vi "After Launch Init.vi"(8 "error in (no error)":errorcluster, 11 "CS++DCPwr in":refnum<class "CS++DCPwr.lvclass">) -> (0 "error out":errorcluster, 3 "CS++DCPwr out":refnum<class "CS++DCPwr.lvclass">)   [LabVIEW 2013, in "CS++DCPwr.lvlib" / "CS++DCPwr.lvclass"]
doc: "Use <b>Pre Launch init.vi</b> method for sanity checks that are supposed to prevent the actor from launching if they fail. Use <B>this</B> method instead to initialize this actor when it has been activated. A corresponding high priority message will become dispatched before the <B>Actor Core.vi</b> is called.\n\nRefer also to the ongoing discussion at https://decibel.ni.com/content/message/57394#57394."
uses:
  CS++DCPwr.lvclass
  Core/Classes/CS++ProcessVariables/SVConnection/SVConnection.lvclass
  CS++DCPwr.lvclass/CS++DCPwr.ctl
  Core/Classes/CS++ProcessVariables/PVConnection/PVConnection.lvclass/PVConnection.ctl
  Core/Actors/CS++DeviceActor/CS++DeviceActor.lvclass
  Core/Actors/CS++DeviceActor/CS++DeviceActor.lvclass/CS++DeviceActor.ctl
  CS++DCPwr Messages/Measure [MSR] Msg/Measure [MSR] Msg.lvclass
  <vilib>/ActorFramework/Actor/Actor.lvclass/Actor.ctl
  <vilib>/ActorFramework/Message Enqueuer/Message Enqueuer.lvclass/Message Enqueuer.ctl
  CS++DCPwr Messages/Measure [MSR] Msg/Measure [MSR] Msg.lvclass/Measure [MSR] Msg.ctl
  CS++DCPwr Messages/Measure [MSR] Msg/Write channel name.vi
  CS++DCPwr Messages/Measure [MSR] Msg/Write measurement type.vi
  <vilib>/ActorFramework/Message Enqueuer/Init from Existing Queue.vi
  <vilib>/ActorFramework/Message Enqueuer/Message Enqueuer.lvclass
  Core/Classes/CS++ProcessVariables/PVConnection/PVConnection.lvclass
  <vilib>/ActorFramework/Actor/Actor.lvclass
  CS++DCPwr Messages/Query Output State Msg/Query Output State Msg.lvclass
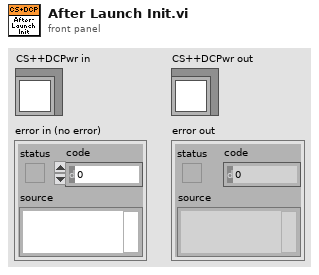
[diagram p1: front panel]
types:
  T1 = cluster{"Write Access":enum8{"Allowed", "Required", "None"}, "Read Access":enum8{"Allowed", "Required", "None"}}
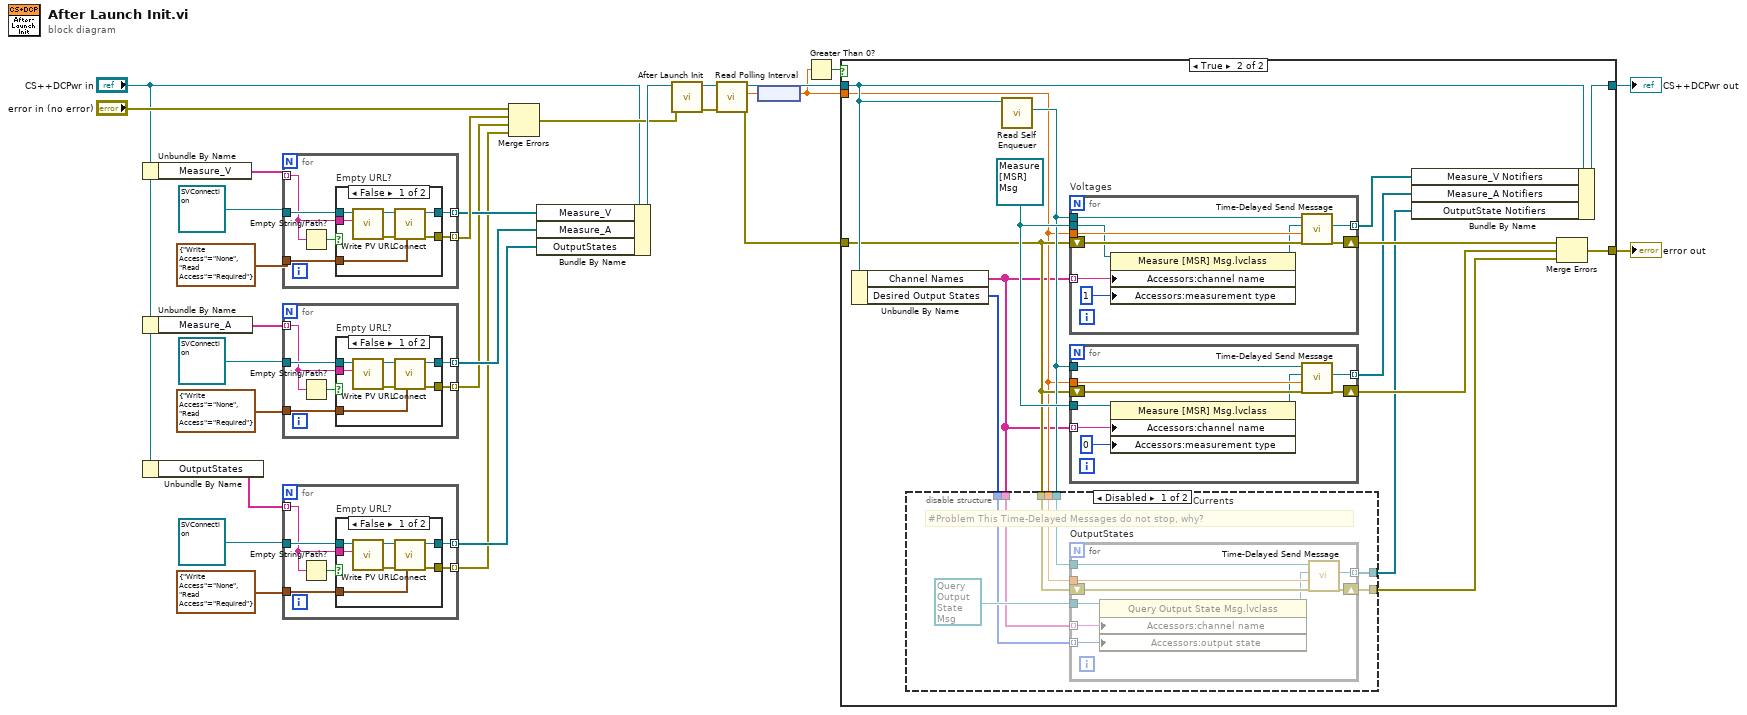
[diagram p0: block diagram]
diagram:
  n1 = Unbundle By Name("CS++DCPwr in") -> ("Measure_V"=w12:string[])
  n2 = Unbundle By Name("CS++DCPwr in") -> ("Measure_A"=w11:string[])
  n3 = Unbundle By Name("CS++DCPwr in") -> ("OutputStates"=w4:string[])
  n4 = for {
    tunnel: w12 -> [w30] mode=indexing
    tunnel: refnum<class "SVConnection.lvclass"> refnum ("CS++ProcessVariables.lvlib:SVConnection.lvclass") -> [w34]
    tunnel: T1 {"Write Access"=enum."None", "Read Access"=enum."Required"} ("Access") -> [w33]
    tunnel: [w32] -> w13 mode=indexing
    tunnel: [w29] -> w24 mode=indexing
    n5 = Empty String/Path?(string/path=w30) -> (empty?=w31:bool)
    n6 = case "Empty URL?" shown="False" w31 {
      tunnel: w34 -> [w41 w42]
      tunnel: w30 -> [w40 _]
      tunnel: w33 -> [w37 _]
      tunnel: [w36 w42] -> w32
      tunnel: [w35 _] -> w29
      frame False {
        n7 = call "Write PV URL.vi"("PV URL"=w40, "PVConnection in"=w41) -> ("error out"=w38:errorcluster, "PVConnection out"=w39:refnum<class "SVConnection.lvclass">)  [unwired: 8 in]
        n8 = call-dynamic "Connect.vi"("Access"=w37, "error in (no error)"=w38, "PVConnection in"=w39) -> ("error out"=w35:errorcluster, "PVConnection out"=w36:refnum<class "SVConnection.lvclass">)  [unwired: 7 in]
      }
      frame True {
      }
    }
  }
  n9 = for {
    tunnel: w11 -> [w44] mode=indexing
    tunnel: refnum<class "SVConnection.lvclass"> refnum ("CS++ProcessVariables.lvlib:SVConnection.lvclass") -> [w48]
    tunnel: T1 {"Write Access"=enum."None", "Read Access"=enum."Required"} ("Access") -> [w47]
    tunnel: [w46] -> w8 mode=indexing
    tunnel: [w43] -> w7 mode=indexing
    n10 = Empty String/Path?(string/path=w44) -> (empty?=w45:bool)
    n11 = case "Empty URL?" shown="False" w45 {
      tunnel: w48 -> [w55 w56]
      tunnel: w44 -> [w54 _]
      tunnel: w47 -> [w51 _]
      tunnel: [w50 w56] -> w46
      tunnel: [w49 _] -> w43
      frame False {
        n12 = call "Write PV URL.vi"("PV URL"=w54, "PVConnection in"=w55) -> ("error out"=w52:errorcluster, "PVConnection out"=w53:refnum<class "SVConnection.lvclass">)  [unwired: 8 in]
        n13 = call-dynamic "Connect.vi"("Access"=w51, "error in (no error)"=w52, "PVConnection in"=w53) -> ("error out"=w49:errorcluster, "PVConnection out"=w50:refnum<class "SVConnection.lvclass">)  [unwired: 7 in]
      }
      frame True {
      }
    }
  }
  n14 = for {
    tunnel: w4 -> [w58] mode=indexing
    tunnel: refnum<class "SVConnection.lvclass"> refnum ("CS++ProcessVariables.lvlib:SVConnection.lvclass") -> [w62]
    tunnel: T1 {"Write Access"=enum."None", "Read Access"=enum."Required"} ("Access") -> [w61]
    tunnel: [w60] -> w2 mode=indexing
    tunnel: [w57] -> w1 mode=indexing
    n15 = Empty String/Path?(string/path=w58) -> (empty?=w59:bool)
    n16 = case "Empty URL?" shown="False" w59 {
      tunnel: w62 -> [w69 w70]
      tunnel: w58 -> [w68 _]
      tunnel: w61 -> [w65 _]
      tunnel: [w64 w70] -> w60
      tunnel: [w63 _] -> w57
      frame False {
        n17 = call "Write PV URL.vi"("PV URL"=w68, "PVConnection in"=w69) -> ("error out"=w66:errorcluster, "PVConnection out"=w67:refnum<class "SVConnection.lvclass">)  [unwired: 8 in]
        n18 = call-dynamic "Connect.vi"("Access"=w65, "error in (no error)"=w66, "PVConnection in"=w67) -> ("error out"=w63:errorcluster, "PVConnection out"=w64:refnum<class "SVConnection.lvclass">)  [unwired: 7 in]
      }
      frame True {
      }
    }
  }
  n19 = Merge Errors("error in (no error)", w24, w7, w1) -> (w25:errorcluster)
  n20 = Bundle By Name(cluster="CS++DCPwr in", "Measure_V"=w13, "Measure_A"=w8, "OutputStates"=w2) -> (w26:refnum<class "CS++DCPwr.lvclass">)
  n21 = call-parent "After Launch Init.vi"("error in (no error)"=w25, "CS++DeviceActor in"=w26) -> ("error out"=w21:errorcluster, "CS++DeviceActor out"=w23:refnum<class "CS++DCPwr.lvclass">)  [unwired: 8 in]
  n22 = call "Read Polling Interval.vi"("error in (no error)"=w21, "CS++DeviceActor in"=w23) -> ("error out"=w20:errorcluster, "Polling Interval"=w19:dbl[unit], "CS++DeviceActor out"=w22:refnum<class "CS++DCPwr.lvclass">)  [unwired: 7 in]
  n23 = node(w19) -> (w18:dbl)
  n24 = Greater Than 0?(x=w18) -> (x > 0?=w17:bool)
  n25 = case shown="True" w17 {
    tunnel: [w72 w87] -> w15
    tunnel: [w71 w85] -> w14
    tunnel: w22 -> [w72 w86]
    tunnel: w20 -> [w71 w78]
    tunnel: w18 -> [_ w77]
    frame False {
    }
    frame True {
      w80 = refnum<class "Measure [MSR] Msg.lvclass"> refnum ("CS++DCPwr.lvlib:Measure [MSR] Msg.lvclass")
      n26 = Unbundle By Name(w86) -> ("Channel Names"=w76:string[], "Desired Output States"=w73:i32[])
      n27 = call <vilib>:"Read Self Enqueuer.vi"("Actor"=w86) -> ("Self Enqueuer"=w79:refnum<class "Message Enqueuer.lvclass">)  [unwired: 10 in]
      n28 = disable-structure shown="Disabled" {
        disable-tunnel: w79 -> [w95 _]
        disable-tunnel: w78 -> [w94 _]
        disable-tunnel: w77 -> [w93 _]
        disable-tunnel: w76 -> [w91 _]
        disable-tunnel: [w90 _] -> w75
        disable-tunnel: [w89 _] -> w74
        disable-tunnel: w73 -> [w88 _]
        frame Disabled {
          # "#Problem This Time-Delayed Messages do not stop, why?"
          n29 = for "OutputStates" {
            tunnel: w95 -> [w103]
            tunnel: w93 -> [w101]
            tunnel: [w100] -> w89 mode=indexing
            shift-right: [w104] -> w90
            shift-left: w94 -> [w102]
            tunnel: w91 -> [w99] mode=indexing
            tunnel: refnum<class "Query Output State Msg.lvclass"> refnum ("CS++DCPwr.lvlib:Query Output State Msg.lvclass") -> [w97]
            tunnel: w88 -> [w96] mode=indexing
            n30 = property class="Query Output State Msg.lvclass"(reference=w97, "Accessors:channel name"=w99, "Accessors:output state"=w96) -> (reference out=w98:refnum<class "Query Output State Msg.lvclass">)  [unwired: 1 in, 1 out]
            n31 = call <vilib>:"Time-Delayed Send Message.vi"("error in (no error)"=w102, "Milliseconds To Wait"=w101, "Message"=w98, "Message Enqueuer"=w103) -> ("error out"=w104:errorcluster, "Delivery Notifier"=w100:refnum<notifier>)  [unwired: 6 in]
          }
        }
        frame Enabled {
        }
      }
      n32 = for "Voltages" {
        tunnel: w79 -> [w121]
        tunnel: w77 -> [w119]
        tunnel: [w118] -> w83 mode=indexing
        tunnel: w80 -> [w114]
        shift-right: [w122] -> w84
        shift-left: w78 -> [w120]
        tunnel: w76 -> [w117] mode=indexing
        n33 = property class="Measure [MSR] Msg.lvclass"(reference=w114, "Accessors:channel name"=w117, "Accessors:measurement type"=1 ("measurement type (voltage)")) -> (reference out=w115:refnum<class "Measure [MSR] Msg.lvclass">)  [unwired: 1 in, 1 out]
        n34 = call <vilib>:"Time-Delayed Send Message.vi"("error in (no error)"=w120, "Milliseconds To Wait"=w119, "Message"=w115, "Message Enqueuer"=w121) -> ("error out"=w122:errorcluster, "Delivery Notifier"=w118:refnum<notifier>)  [unwired: 6 in]
      }
      n35 = for "Currents" {
        tunnel: w79 -> [w112]
        tunnel: w77 -> [w110]
        tunnel: [w109] -> w82 mode=indexing
        shift-right: [w113] -> w81
        shift-left: w78 -> [w111]
        tunnel: w76 -> [w108] mode=indexing
        tunnel: w80 -> [w105]
        n36 = property class="Measure [MSR] Msg.lvclass"(reference=w105, "Accessors:channel name"=w108, "Accessors:measurement type"=0 ("measurement type (voltage)")) -> (reference out=w106:refnum<class "Measure [MSR] Msg.lvclass">)  [unwired: 1 in, 1 out]
        n37 = call <vilib>:"Time-Delayed Send Message.vi"("error in (no error)"=w111, "Milliseconds To Wait"=w110, "Message"=w106, "Message Enqueuer"=w112) -> ("error out"=w113:errorcluster, "Delivery Notifier"=w109:refnum<notifier>)  [unwired: 6 in]
      }
      n38 = Bundle By Name(cluster=w86, "Measure_V Notifiers"=w83, "Measure_A Notifiers"=w82, "OutputState Notifiers"=w74) -> (w87:refnum<class "CS++DCPwr.lvclass">)
      n39 = Merge Errors(w84, w81, w75) -> (w85:errorcluster)
    }
  }
  "error out" <- w14
  "CS++DCPwr out" <- w15
